vi "StopCapture.vi"(8 "error in (no error)":errorcluster, 11 "ZWO_ASI in":refnum<class "ZWO_ASI.lvclass">) -> (0 "error out":errorcluster, 3 "ZWO_ASI out":refnum<class "ZWO_ASI.lvclass">)   [LabVIEW 2023, in "ZWO_ASI.lvlib" / "ZWO_ASI.lvclass"]
uses:
  ZWO_ASI.lvclass
  ZWO_ASI.lvclass/ZWO_ASI.ctl
  <userlib>/ASICamera2_no_err/ASICamera2_no_err.lvlib
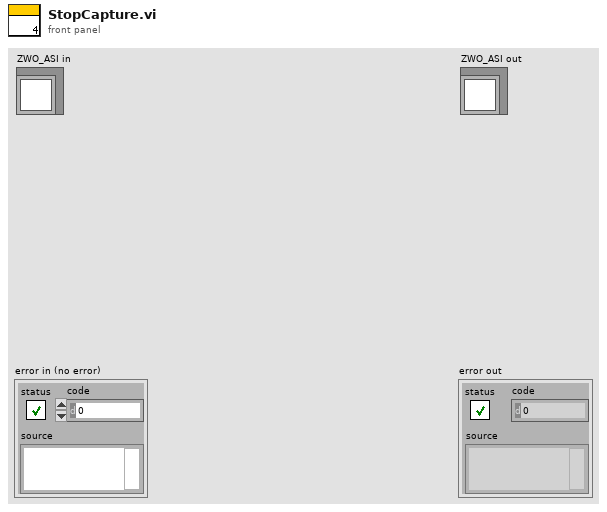
[diagram p1: front panel]
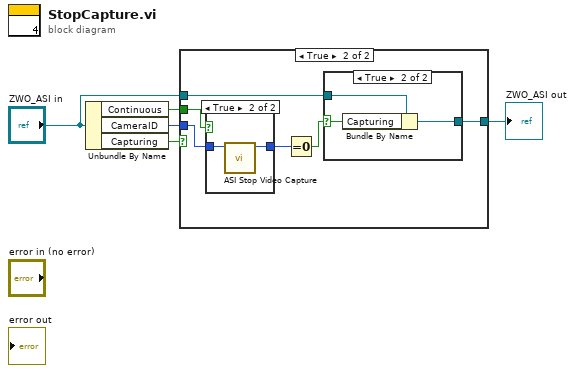
[diagram p0: block diagram]
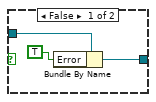
[diagram p3: hidden frame]
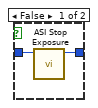
[diagram p4: hidden frame]
diagram:
  n1 = Unbundle By Name("ZWO_ASI in") -> ("Continuous"=w4:bool, "CameraID"=w3:i32, "Capturing"=w2:bool)
  n2 = case shown="True" w2 {
    tunnel: "ZWO_ASI in" -> [w6 w10]
    tunnel: w4 -> [_ w9]
    tunnel: w3 -> [_ w8]
    tunnel: [w6 w7] -> w1
    frame False {
    }
    frame True {
      n3 = case shown="True" w9 {
        tunnel: [w19 w21] -> w12
        tunnel: w8 -> [w20 w22]
        frame False {
          n4 = call <userlib>:"ASI Stop Exposure.vi"("iCameraID"=w20) -> ("function return"=w19:i32)  [unwired: 10 in]
        }
        frame True {
          n5 = call <userlib>:"ASI Stop Video Capture.vi"("iCameraID"=w22) -> ("function return"=w21:i32)  [unwired: 10 in]
        }
      }
      n6 = Equal To 0?(x=w12) -> (x = 0?=w11:bool)
      n7 = case shown="True" w11 {
        selector: w11 -> [_ w18]
        tunnel: w10 -> [w15 w17]
        tunnel: [w14 w16] -> w7
        frame False {
          n8 = Bundle By Name(cluster=w15, "Error"=TRUE) -> (w14:refnum<class "ZWO_ASI.lvclass">)
        }
        frame True {
          n9 = Bundle By Name(cluster=w17, "Capturing"=w18) -> (w16:refnum<class "ZWO_ASI.lvclass">)
        }
      }
    }
  }
  "ZWO_ASI out" <- w1
